vi "UTIL_Quit LabVIEW if Executable v1_0_0.vi"(7 "error in (no error)":errorcluster) -> (0 "error out":errorcluster)   [LabVIEW 2015]
doc: "UTIL_Quit LabVIEW if Executable v1_0_0.vi\n\nChecks the current path to this VI to see if it is called as part of an executable. If the caller of this sub-vi is the top level in the vi hierachy, the \"Quit LabVIEW\" VI is called.\n\nDeveloped by:\n J. Daren Suntych\nNational Analytics 2006\n970-397-0764"
panel:
  # "Checks the current path to this VI to see if it\nis called as part of an executable.  If so, the\n\"Quit LabVIEW\" VI is called."
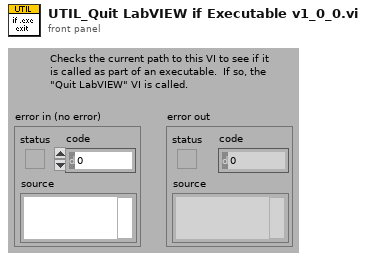
[diagram p1: front panel]
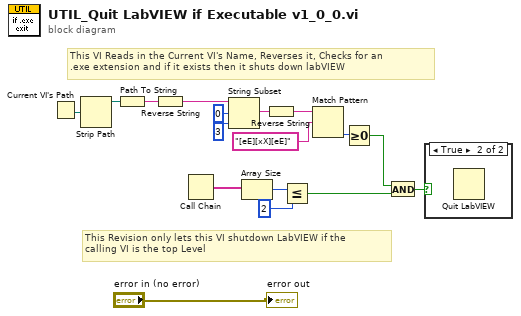
[diagram p0: block diagram]
diagram:
  # "This Revision only lets this VI shutdown LabVIEW if the \ncalling VI is the top Level"
  # "This VI Reads in the Current VI's Name, Reverses it, Checks for an\n.exe extension and if it exists then it shuts down labVIEW"
  n1 = Current VI's Path() -> (path=w17:path)
  n2 = Strip Path(path=w17) -> (stripped path=w8:path)  [unwired: 1 out]
  n3 = Path To String(path=w8) -> (string=w16:string)
  n4 = Reverse String(1:w16) -> (0:w15:string)
  n5 = Call Chain() -> (call chain=w6:string[])
  n6 = String Subset(string=w15, offset (0)=0, length (rest)=3 ("length")) -> (substring=w12:string)
  n7 = Array Size(array=w6) -> (size(s)=w5:i32)
  n8 = Reverse String(1:w12) -> (0:w11:string)
  n9 = Less Or Equal?(x=w5, y=2) -> (x <= y?=w3:bool)
  n10 = Match Pattern(string=w11, regular expression="[eE][xX][eE]") -> (offset past match=w9:i32)  [unwired: 4 out]
  n11 = Greater Or Equal To 0?(x=w9) -> (x >= 0?=w2:bool)
  n12 = And(x=w2, y=w3) -> (x .and. y?=w1:bool)
  n13 = case shown="True" w1 {
    frame False {
    }
    frame True {
      n14 = Quit LabVIEW() -> ()  [unwired: 1 out]
    }
  }
  "error out" <- "error in (no error)"
